vi "Migrate Shared Dependencies.vi"(0 "Project path":path, 5 "Measurement path":path, 7 "Common dependencies":path[](array[path]), 11 "error in (no error)":errorcluster) -> (4 "Outside items":string[](array[string]), 15 "error out":errorcluster)   [LabVIEW 2021]
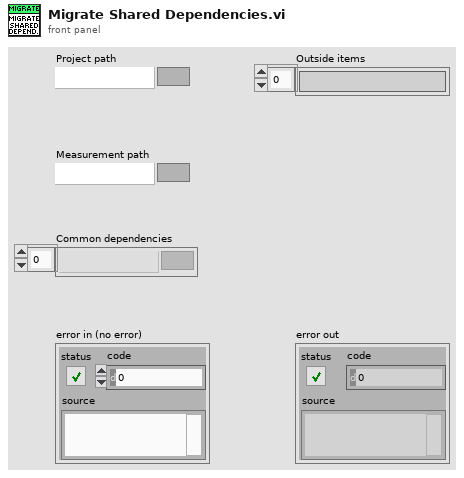
[diagram p1: front panel]
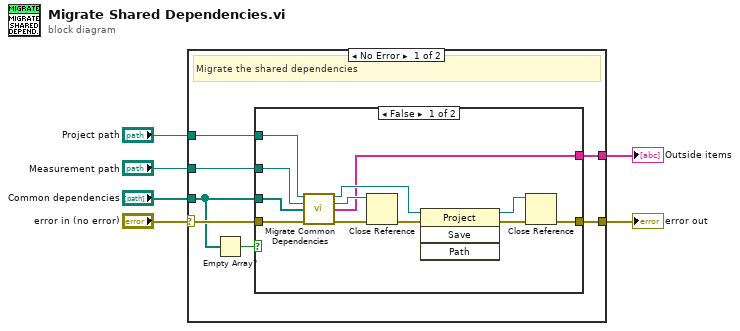
[diagram p0: block diagram]
diagram:
  n1 = case shown="No Error" "error in (no error)" {
    selector: "error in (no error)" -> [w12 w27]
    tunnel: [w13 w27] -> w6
    tunnel: "Common dependencies" -> [w9 _]
    tunnel: "Project path" -> [w11 _]
    tunnel: [w10 _] -> w2
    tunnel: "Measurement path" -> [w7 _]
    frame No Error {
      # "Migrate the shared dependencies"
      n2 = Empty Array?(array=w9) -> (empty?=w8:bool)
      n3 = case shown="False" w8 {
        tunnel: w12 -> [w25 w26]
        tunnel: [w21 w26] -> w13
        tunnel: w9 -> [w17 _]
        tunnel: w11 -> [w16 _]
        tunnel: [w15 _] -> w10
        tunnel: w7 -> [w14 _]
        frame False {
          n4 = call "Migrate Common Dependencies.vi"("Project path"=w16, "Measurement path"=w14, "Dependencies path"=w17, "error in (no error)"=w25) -> ("Project reference"=w19:refnum<vi>, "MeasurementCore reference"=w22:refnum<vi>, "Outside items"=w15:string[], "error out"=w24:errorcluster)  [unwired: 8 in]
          n5 = Close Reference(reference=w22, error in (no error)=w24) -> (error out=w23:errorcluster)
          n6 = invoke class="Project" method="Save"(reference=w19, error in=w23) -> (reference out=w18:refnum<vi>, error out=w20:errorcluster)  [unwired: 2 in, 2 out]
          n7 = Close Reference(reference=w18, error in (no error)=w20) -> (error out=w21:errorcluster)
        }
        frame True {
        }
      }
    }
    frame Error {
      # "Pass"
    }
  }
  "error out" <- w6
  "Outside items" <- w2
